vi "ConvertStrToBool.vi"(11 "bool str":string) -> (3 "result":bool)   [LabVIEW 2018, in "Library-DataConvert.lvlib"]
uses:
  Library-DataConvert.lvlib
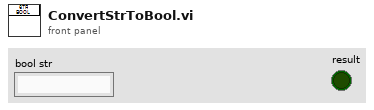
[diagram p1: front panel]
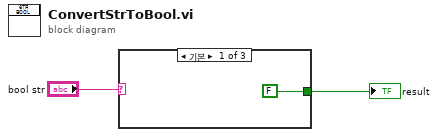
[diagram p0: block diagram]
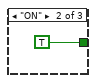
[diagram p2: hidden frame]
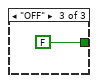
[diagram p3: hidden frame]
diagram:
  n1 = case shown="기본" "bool str" {
    tunnel: [FALSE TRUE FALSE] -> w1
    frame Default {
    }
    frame "ON" {
    }
    frame "OFF" {
    }
  }
  "result" <- w1
